vi "Is Entity Cached.vi"(8 "error in (no error)":errorcluster, 10 "Entity":refnum<class "Entity.lvclass">, 11 "Unit Of Work in":refnum<class "Unit Of Work Session.lvclass">) -> (0 "error out":errorcluster, 2 "Cached":bool)   [LabVIEW 2020, in "Conditu2.lvlib" / "Unit Of Work Session.lvclass"]
uses:
  Unit Of Work Session.lvclass
  Entity/Entity.lvclass
  Unit Of Work Session.lvclass/Unit Of Work Session.ctl
  Entity/Entity.lvclass/Entity.ctl
  Columns/ID/ID.lvclass/ID.ctl
  Columns/ID/Get.vi
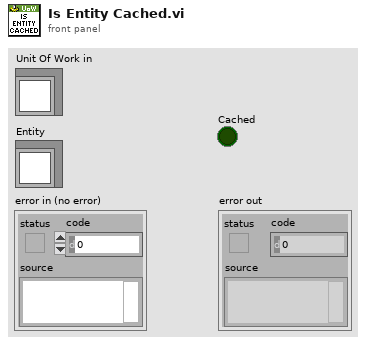
[diagram p1: front panel]
types:
  T1 = typedef "Conditu2.lvlib/Entity ID.ctl" = i64
  T2 = typedef "Conditu2.lvlib/Unit Of Work Session.lvclass/Ref Data.ctl" = cluster{"Entity Class Map":T3}
  T3 = typedef "Conditu2.lvlib/Unit Of Work Session.lvclass/Entity Class Map.ctl" = map{string, map{T1, refnum<class "Entity.lvclass">}}
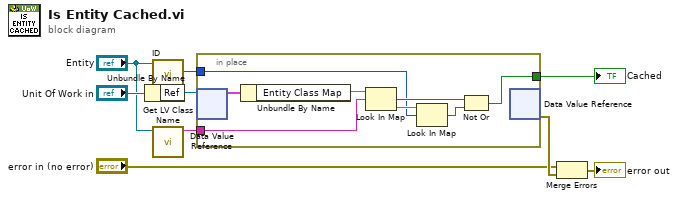
[diagram p0: block diagram]
diagram:
  n1 = Unbundle By Name("Unit Of Work in") -> ("Ref"=w8:refnum<data-value>)
  n2 = call "ID.vi"("Entity in"="Entity") -> ("ID"=w5:T1)  [unwired: 9 in, 1 out]
  n3 = call <vilib>:"Get LV Class Name.vi"("object"="Entity") -> ("class name"=w9:string)  [unwired: 9 in, 1 out]
  n4 = in-place {
    in-place-border: w9 -> [w16]
    in-place-border: w5 -> [w11]
    in-place-border: [w10] -> w4
    n5 = in-place-dvr #1(w8) -> (w17:T2)  [unwired: 1 out]
    n6 = Unbundle By Name(w17) -> ("Entity Class Map"=w15:T3)
    n7 = Look In Map(map=w15, key=w16) -> (key not found?=w13:bool, value=w14:map{T1, refnum<class "Entity.lvclass">})  [unwired: 1 in]
    n8 = Look In Map(map=w14, key=w11) -> (key not found?=w12:bool)  [unwired: 1 in, 1 out]
    n9 = Not Or(1:w12, 2:w13) -> (0:w10:bool)
    n10 = in-place-dvr #1() -> (w3:errorcluster)  [unwired: 1 in, 1 out]
  }
  "Cached" <- w4
  n11 = Merge Errors("error in (no error)", w3) -> (→"error out":errorcluster)
